vi "Module for RF and LO synthesizer.vi"(10 "Main controller mailbox":T3, 11 "THz module mailbox":T3) -> ()   [LabVIEW 2024, in "THz source modeule.lvlib"]
doc: "Module to set constant frequency or simple frequency sweep on RF (main) synthesizer and offset frequency on LO (folowing) synthesizer.\nKey typedefs: THz_Message for module, THz_Comands enum (Ignore, Initialize, Update, Set parameters, Disconnect, End), THz_Sweeep parameters\n\nComands and responses:\nInitialize: VDI config constants {Master{lower limit, upper limit, name, handle, description}, Follower{ lower limit, upper limit, name, handle, description } } (cluster of two clusters {numeric, numeric, string, numeric, string}) / handle log (string)\nUpdate: - / M_ID F_ID (string)\nSet parameters: Sweep parameters {Start, End, Sweep up time, Sweep down time, Intermediate, Reset trigger} (cluster{numeric, numeric, numeric, numeric, numeric, boolean}) / Sweep parameters (same cluster)\nDisconnect: - / master and follower name (string)\nEnd: - / Master and Follower handle (string)"
uses:
  THz source modeule.lvlib
  Messenger service/Data types/Mailbox address.ctl
  ctl/THz MW generator constants.ctl
  ctl/THz sweep parameters.ctl
  Messenger service/Data types/Module name.ctl
  ctl/THz Message for module.ctl
  ctl/THz commands enum.ctl
  <vilib>/Utility/error.llb/Error Cluster From Error Code.vi
  <vilib>/ErrorRing/Error Ring.xnode
  Messenger service/MessengerLib.lvlib
panel:
  out "FT_Status_Update_Master":u32(ring) items=["FT_OK", "FT_INVALID_HANDLE", "FT_DEVICE_NOT_FOUND", "FT_DEVICE_NOT_OPENED", "FT_IO_ERROR", "FT_INSUFFICIENT_RESOURCES", "FT_INVALID_PARAMETER", "FT_INVALID_BAUD_RATE", "FT_DEVICE_NOT_OPENED_FOR_ERASE", "FT_DEVICE_NOT_OPENED_FOR_WRITE", "FT_FAILED_TO_WRITE_DEVICE", "FT_EEPROM_READ_FAILED", "FT_EEPROM_WRITE_FAILED", "FT_EEPROM_ERASE_FAILED", "FT_EEPROM_NOT_PRESENT", "FT_EEPROM_NOT_PROGRAMMED", "FT_INVALID_ARGS", "FT_NOT_SUPPORTED", "FT_OTHER_ERROR"]
  out "Sweep parameters":T1={"Start [GHz]"=8.0, "End [GHz] "=8.0, "Sweep up\ntime [ms]"=0.0, "Sweep down\ntime [ms]"=0.0, "Intermidiate [MHz]"=0.0, "Reset trigger"=FALSE} {"Sweep down\ntime [ms]" min=0.0 max=250.0; "End [GHz]" min=8.0 max=20.0; "Intermidiate [MHz]" min=0.0 max=2500.0; "Start [GHz]" min=8.0 max=20.0}
  out "FT_Status Update F":u32(ring) items=["FT_OK", "FT_INVALID_HANDLE", "FT_DEVICE_NOT_FOUND", "FT_DEVICE_NOT_OPENED", "FT_IO_ERROR", "FT_INSUFFICIENT_RESOURCES", "FT_INVALID_PARAMETER", "FT_INVALID_BAUD_RATE", "FT_DEVICE_NOT_OPENED_FOR_ERASE", "FT_DEVICE_NOT_OPENED_FOR_WRITE", "FT_FAILED_TO_WRITE_DEVICE", "FT_EEPROM_READ_FAILED", "FT_EEPROM_WRITE_FAILED", "FT_EEPROM_ERASE_FAILED", "FT_EEPROM_NOT_PRESENT", "FT_EEPROM_NOT_PROGRAMMED", "FT_INVALID_ARGS", "FT_NOT_SUPPORTED", "FT_OTHER_ERROR"]
  out "Ended":bool
  out "Constants":T2[](array[typedef])=[{"Lower limit [GHz]"=9.0, "Upper limit [GHz]"=15.0, "Device name"="VDIS0122", "Connection"="0", "Description"="VDI Synth", "Connected"=FALSE, "Last settings"="", "Operation mode"=enum."Disabled", "Enable ch 1"=FALSE, "Enable ch 2"=FALSE}, {"Lower limit [GHz]"=0.01, "Upper limit [GHz]"=1.3, "Device name"="VDIYT7", "Connection"="0", "Description"="VDI Tracking", "Connected"=FALSE, "Last settings"="", "Operation mode"=enum."Disabled", "Enable ch 1"=FALSE, "Enable ch 2"=FALSE}]
  out "Connected":bool
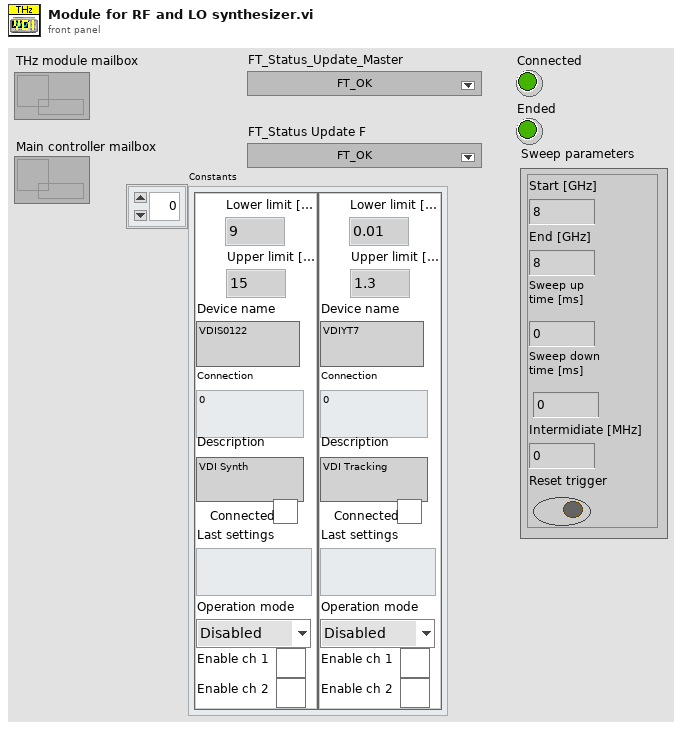
[diagram p1: front panel]
types:
  T1 = typedef "THz source modeule.lvlib/THz sweep parameters.ctl" = cluster{"Start [GHz]":dbl, "End [GHz] ":dbl, "Sweep up\ntime [ms]":dbl, "Sweep down\ntime [ms]":dbl, "Intermidiate [MHz]":dbl, "Reset trigger":bool}
  T2 = typedef "THz source modeule.lvlib/THz MW generator constants.ctl" = cluster{"Lower limit [GHz]":dbl, "Upper limit [GHz]":dbl, "Device name":string, "Connection":string, "Description":string, "Connected":bool, "Last settings":string, "Operation mode":enum16{"Disabled", "CW", "Arbitrary", "Sweep"}, "Enable ch 1":bool, "Enable ch 2":bool}
  T3 = typedef "MessengerLib.lvlib/Mailbox address.ctl" = refnum<queue>
  T4 = typedef "THz source modeule.lvlib/THz Message for module.ctl" = cluster{"Command":T5, "Data":variant}
  T5 = typedef "THz source modeule.lvlib/THz commands enum.ctl" = enum16{"Ignore", "Connect", "Update", "Set parameters", "Disconnect", "End"}
  T6 = typedef "Module name.ctl" = enum16{"Emty", "Magnet", "VTI", "Excitation", "Servo", "Acquisition", "Rotator", "Digitizer", "SMU2450", "Carousel", "Multimeter", "Tmp monitor", "Power monitor"}
  T7 = typedef "THz source modeule.lvlib/VDI status.ctl" = cluster{"Master":T8, "Follower":T8}
  T8 = typedef "THz source modeule.lvlib/Synth status.ctl" = cluster{"Mode":enum16{"CW", "Sweep"}, "Conected":bool}
  T9 = cluster{"Type":u32, "VID":string, "PID":string, "Serial Number":string, "Description":string}
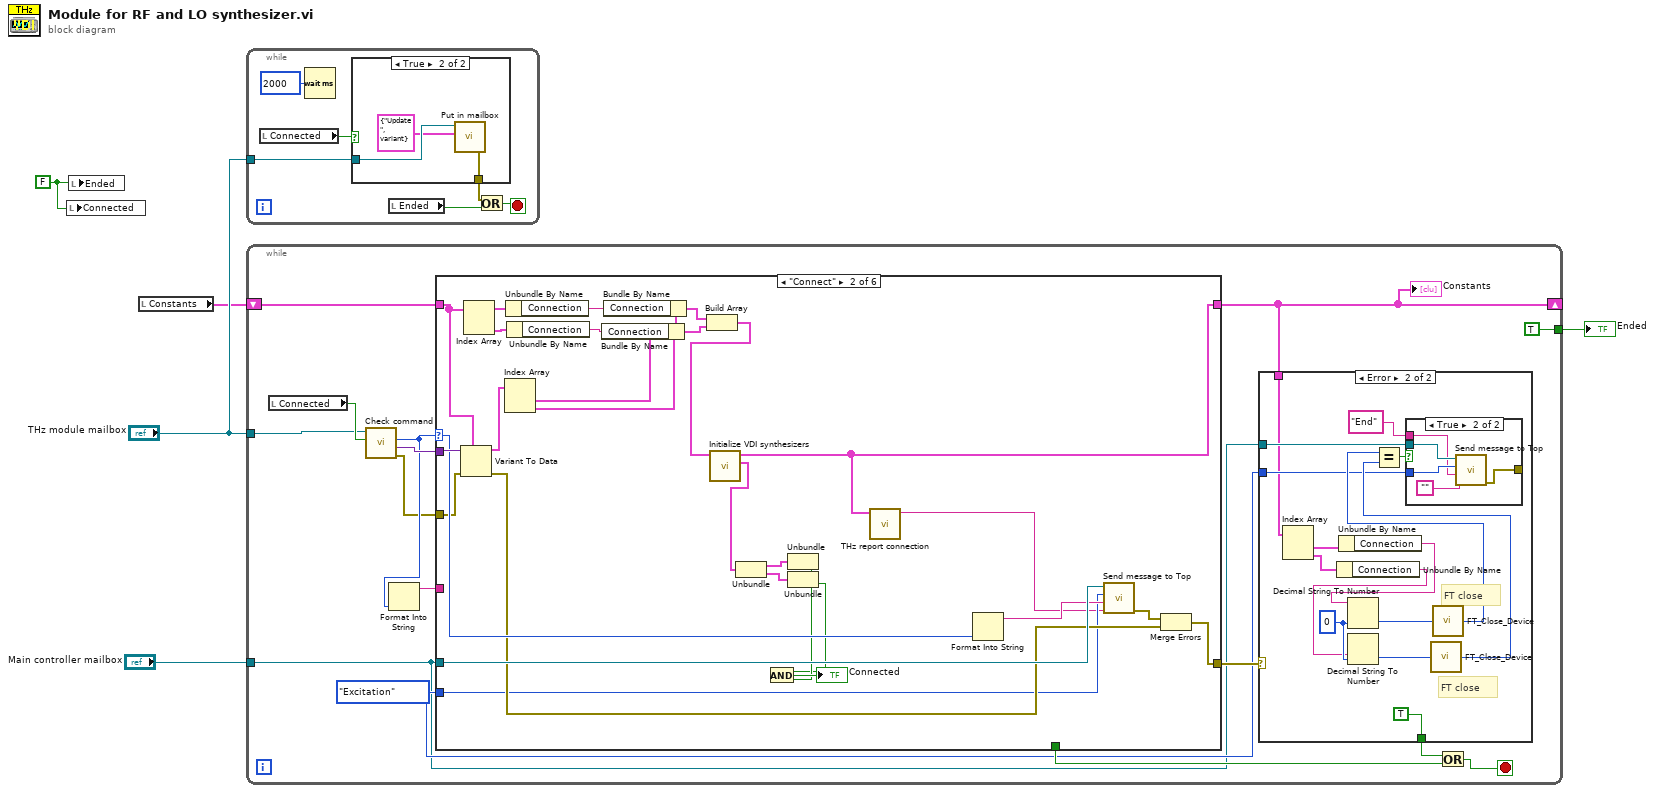
[diagram p0: block diagram]
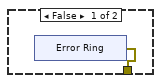
[diagram p2: hidden frame]
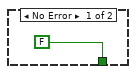
[diagram p3: hidden frame]
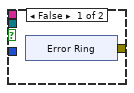
[diagram p4: hidden frame]
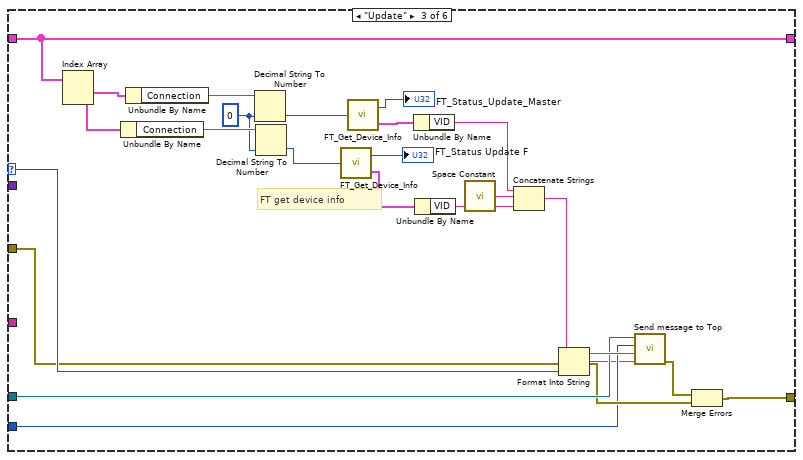
[diagram p6: hidden frame]
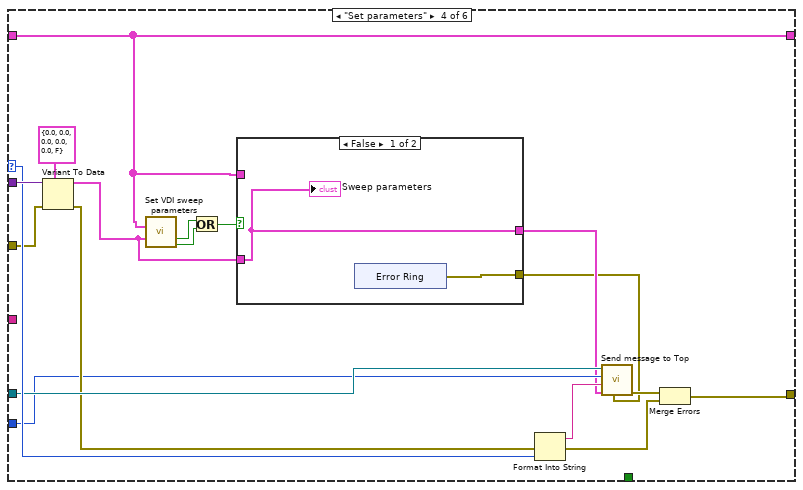
[diagram p7: hidden frame]
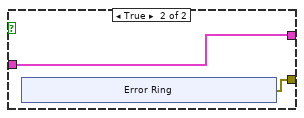
[diagram p8: hidden frame]
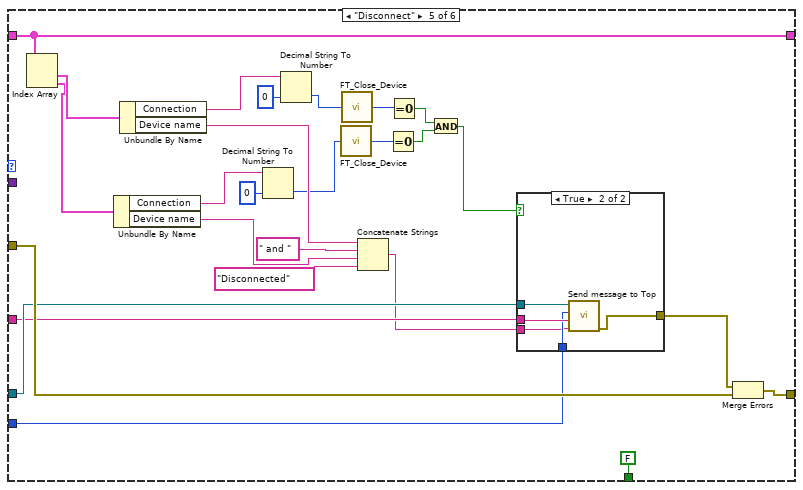
[diagram p9: hidden frame]
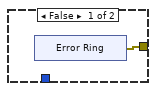
[diagram p10: hidden frame]
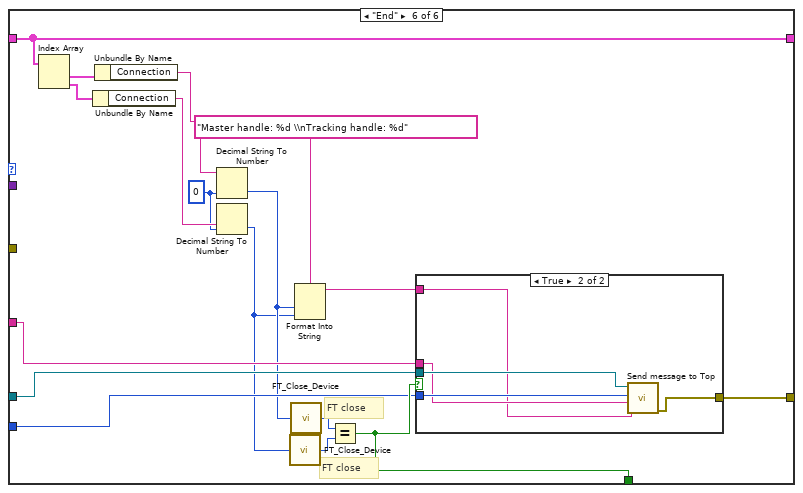
[diagram p11: hidden frame]
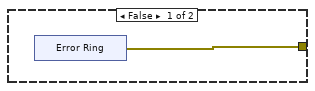
[diagram p12: hidden frame]
diagram:
  w1 = FALSE ("Initialized")
  n1 = local write "Connected"(w1) -> ()
  n2 = local write "Ended"(w1) -> ()
  n3 = local read "Constants"() -> (w3:T2[])
  n4 = while {
    tunnel: "THz module mailbox" -> [w9]
    stop <- w8 stop-if-true
    n5 = local read "Connected"() -> (w10:bool)
    n6 = Wait (ms)(milliseconds to wait=u32 2000) -> ()  [unwired: 1 out]
    n7 = case shown="True" w10 {
      tunnel: w9 -> [_ w16]
      tunnel: [w12 w14] -> w7
      frame False {
        n8 = xnode "Error Ring"() -> ("error out"=w12:errorcluster)
      }
      frame True {
        n9 = call "Put in mailbox.vi"("Message"=T4 {"Command"=enum."Update", "Data"=variant} ("Incoming msg"), "Queue in"=w16) -> ("error out"=w14:errorcluster)  [unwired: 7 in, 2 out]
      }
    }
    n10 = local read "Ended"() -> (w6:bool)
    n11 = Or(x=w7, y=w6) -> (x .or. y?=w8:bool)
  }
  n12 = while {
    shift-right: [w28] -> _
    shift-left: w3 -> [w31]
    tunnel: "THz module mailbox" -> [w20]
    tunnel: "Main controller mailbox" -> [w17]
    tunnel: [TRUE ("Initialized")] -> w2
    stop <- w26 stop-if-true
    w18 = Module_name."Excitation" ("Module")
    n13 = local read "Connected"() -> (w29:bool)
    n14 = call "Check command.vi"("Is connected"=w29, "Module mailbox"=w20) -> ("error out"=w19:errorcluster, "Command Data"=w30:variant, "Command"=w22:T5)  [unwired: 3 in]
    n15 = Format Into String(w22) -> (resulting string=w21:string)  [unwired: 3 in, 1 out]
    n16 = case shown="\"Connect\"" w22 {
      selector: w22 -> [_ w83 w107 w123 _ _]
      tunnel: [w56 w58 w101 w109 w158 w172] -> w28
      tunnel: w31 -> [w56 w71 w101 w109 w158 w172]
      tunnel: w30 -> [_ w84 _ w126 _ _]
      tunnel: [_ _ _ _ FALSE w184] -> w27
      tunnel: w17 -> [_ w82 w106 w121 w157 w185]
      tunnel: [w55 w78 w104 w117 w160 w183] -> w23
      tunnel: w19 -> [w55 w76 w103 w119 w161 _]
      tunnel: w18 -> [_ w72 w100 w114 w150 w179]
      tunnel: w21 -> [_ _ _ _ w151 w182]
      frame "Ignore", Default {
      }
      frame "Connect" {
        n17 = Variant To Data(error in=w76, type=w71, Variant=w84) -> (data=w68:T2[], error out=w75:errorcluster)
        n18 = Index Array(array=w71) -> (element #1=w70:T2, element #2=w69:T2)  [unwired: 2 in]
        n19 = Index Array(array=w68) -> (element #1=w67:T2, element #2=w63:T2)  [unwired: 2 in]
        n20 = Unbundle By Name(w70) -> ("Connection"=w66:string)
        n21 = Unbundle By Name(w69) -> ("Connection"=w61:string)
        n22 = Bundle By Name(cluster=w63, "Connection"=w61) -> (w62:T2)
        n23 = Bundle By Name(cluster=w67, "Connection"=w66) -> (w64:T2)
        n24 = Build Array(w64, w62) -> (w65:T2[])
        n25 = call "Initialize VDI synthesizers.vi"("VDI config constants in"=w65) -> ("Status"=w74:T7, "VDI config constants out"=w58:T2[])  [unwired: 9 in]
        n26 = Unbundle(w74) -> ("Master"=w79:T8, "Follower"=w73:T8)
        n27 = Unbundle(w79) -> ("Conected"=w60:bool)  [unwired: 1 out]
        n28 = Unbundle(w73) -> ("Conected"=w59:bool)  [unwired: 1 out]
        n29 = And(x=w59, y=w60) -> (x .and. y?=→"Connected":bool)
        n30 = call "THz report connection.vi"("THz MW generator constants"=w58) -> ("string out"=w57:string)  [unwired: 10 in]
        n31 = Format Into String(w83) -> (resulting string=w81:string)  [unwired: 3 in, 1 out]
        n32 = call "Send message to Top.vi"("Data"=w57, "Response"=w81, "Module"=w72, "Mailbox address in"=w82) -> ("Error out"=w77:errorcluster)  [unwired: 6 in, 1 out]
        n33 = Merge Errors(w77, w75) -> (w78:errorcluster)
      }
      frame "Update" {
        w87 = u32 0 ("default (0 I32)")
        # "FT get device info"
        n34 = Index Array(array=w101) -> (element #1=w88:T2, element #2=w89:T2)  [unwired: 2 in]
        n35 = Unbundle By Name(w89) -> ("Connection"=w90:string)
        n36 = Unbundle By Name(w88) -> ("Connection"=w91:string)
        n37 = Decimal String To Number(string=w91, default (0L)=w87) -> (number=w86:u32)  [unwired: 1 in, 1 out]
        n38 = Decimal String To Number(string=w90, default (0L)=w87) -> (number=w85:u32)  [unwired: 1 in, 1 out]
        n39 = call <instrlib>:"FT_Get_Device_Info.vi"("Handle"=w85) -> ("FT_Status"=→"FT_Status Update F":u32, "Device Information"=w99:T9)
        n40 = call <instrlib>:"FT_Get_Device_Info.vi"("Handle"=w86) -> ("FT_Status"=→"FT_Status_Update_Master":u32, "Device Information"=w97:T9)
        n41 = Unbundle By Name(w97) -> ("VID"=w95:string)
        n42 = Unbundle By Name(w99) -> ("VID"=w98:string)
        n43 = call <vilib>:"Space Constant.vi"() -> ("String"=w94:string)
        n44 = Concatenate Strings(w95, w94, w98) -> (w96:string)
        n45 = Format Into String(error in=w103, w107) -> (resulting string=w108:string, error out=w102:errorcluster)  [unwired: 2 in]
        n46 = call "Send message to Top.vi"("Data"=w96, "Response"=w108, "Module"=w100, "Mailbox address in"=w106) -> ("Error out"=w105:errorcluster)  [unwired: 6 in, 1 out]
        n47 = Merge Errors(w105, w102) -> (w104:errorcluster)
      }
      frame "Set parameters" {
        n48 = Variant To Data(error in=w119, type=T1 {"Start [GHz]"=0.0, "End [GHz] "=0.0, "Sweep up\ntime [ms]"=0.0, "Sweep down\ntime [ms]"=0.0, "Intermidiate [MHz]"=0.0, "Reset trigger"=FALSE} ("Sweep parameters"), Variant=w126) -> (data=w111:T1, error out=w118:errorcluster)
        n49 = call "Set VDI sweep parameters.vi"("MW generator constants"=w109, "Sweep parameters"=w111) -> ("Error1"=w122:bool, "Error2"=w120:bool)  [unwired: 9 in, 3 out]
        n50 = Or(x=w122, y=w120) -> (x .or. y?=w113:bool)
        n51 = case shown="False" w113 {
          tunnel: [w128 w130] -> w112
          tunnel: w111 -> [w128 w130]
          tunnel: w109 -> [_ _]
          tunnel: [w127 w131] -> w110
          frame False {
            n52 = xnode "Error Ring"() -> ("error out"=w127:errorcluster)
            "Sweep parameters" <- w128
          }
          frame True {
            n53 = xnode "Error Ring"() -> ("error out"=w131:errorcluster)
          }
        }
        n54 = Format Into String(error in=w118, w123) -> (resulting string=w124:string, error out=w116:errorcluster)  [unwired: 2 in]
        n55 = call "Send message to Top.vi"("Error in (no error)"=w110, "Data"=w112, "Response"=w124, "Module"=w114, "Mailbox address in"=w121) -> ("Error out"=w115:errorcluster)  [unwired: 5 in, 1 out]
        n56 = Merge Errors(w115, w116) -> (w117:errorcluster)
      }
      frame "Disconnect" {
        n57 = Index Array(array=w158) -> (element #1=w143:T2, element #2=w141:T2)  [unwired: 2 in]
        n58 = Unbundle By Name(w141) -> ("Connection"=w136:string, "Device name"=w142:string)
        n59 = Unbundle By Name(w143) -> ("Connection"=w159:string, "Device name"=w149:string)
        n60 = Decimal String To Number(string=w136, default (0L)=u32 0 ("default (0 I32)")) -> (number=w137:u32)  [unwired: 1 in, 1 out]
        n61 = Decimal String To Number(string=w159, default (0L)=u32 0 ("default (0 I32)")) -> (number=w140:u32)  [unwired: 1 in, 1 out]
        n62 = call <instrlib>:"FT_Close_Device.vi"("Handle"=w137) -> ("FT_Status"=w155:u32)
        n63 = call <instrlib>:"FT_Close_Device.vi"("Handle"=w140) -> ("FT_Status"=w154:u32)
        n64 = Concatenate Strings(w149, " and " ("string"), w142, "Disconnected" ("string")) -> (w144:string)
        n65 = Equal To 0?(x=w155) -> (x = 0?=w156:bool)
        n66 = Equal To 0?(x=w154) -> (x = 0?=w153:bool)
        n67 = And(x=w153, y=w156) -> (x .and. y?=w152:bool)
        n68 = case shown="True" w152 {
          tunnel: w157 -> [_ w168]
          tunnel: [w162 w167] -> w146
          tunnel: w151 -> [_ w166]
          tunnel: w150 -> [_ w165]
          tunnel: w144 -> [_ w164]
          frame False {
            n69 = xnode "Error Ring"() -> ("error out"=w162:errorcluster)
          }
          frame True {
            n70 = call "Send message to Top.vi"("Data"=w164, "Response"=w166, "Module"=w165, "Mailbox address in"=w168) -> ("Error out"=w167:errorcluster)  [unwired: 6 in, 1 out]
          }
        }
        n71 = Merge Errors(w146, w161) -> (w160:errorcluster)
      }
      frame "End" {
        w173 = u32 0 ("default (0 I32)")
        # "FT close"
        # "FT close"
        n72 = Index Array(array=w172) -> (element #1=w174:T2, element #2=w175:T2)  [unwired: 2 in]
        n73 = Unbundle By Name(w175) -> ("Connection"=w176:string)
        n74 = Unbundle By Name(w174) -> ("Connection"=w171:string)
        n75 = Decimal String To Number(string=w171, default (0L)=w173) -> (number=w170:u32)  [unwired: 1 in, 1 out]
        n76 = Decimal String To Number(string=w176, default (0L)=w173) -> (number=w169:u32)  [unwired: 1 in, 1 out]
        n77 = call <instrlib>:"FT_Close_Device.vi"("Handle"=w169) -> ("FT_Status"=w180:u32)
        n78 = call <instrlib>:"FT_Close_Device.vi"("Handle"=w170) -> ("FT_Status"=w181:u32)
        n79 = Format Into String(format string="Master handle: %d \\nTracking handle: %d", w170, w169) -> (resulting string=w177:string)  [unwired: 2 in, 1 out]
        n80 = Equal?(x=w181, y=w180) -> (x = y?=w184:bool)
        n81 = case shown="True" w184 {
          tunnel: w185 -> [_ w192]
          tunnel: [w186 w191] -> w183
          tunnel: w179 -> [_ w190]
          tunnel: w182 -> [_ w189]
          tunnel: w177 -> [_ w188]
          frame False {
            n82 = xnode "Error Ring"() -> ("error out"=w186:errorcluster)
          }
          frame True {
            n83 = call "Send message to Top.vi"("Data"=w188, "Response"=w189, "Module"=w190, "Mailbox address in"=w192) -> ("Error out"=w191:errorcluster)  [unwired: 6 in, 1 out]
          }
        }
      }
    }
    "Constants" <- w28
    n84 = case shown="Error" w23 {
      tunnel: w28 -> [_ w40]
      tunnel: [FALSE TRUE] -> w25
      tunnel: w18 -> [_ w42]
      tunnel: w17 -> [_ w41]
      frame No Error {
      }
      frame Error {
        w39 = u32 0 ("default (0 I32)")
        # "FT close"
        # "FT close"
        n85 = Index Array(array=w40) -> (element #1=w38:T2, element #2=w37:T2)  [unwired: 2 in]
        n86 = Unbundle By Name(w37) -> ("Connection"=w36:string)
        n87 = Unbundle By Name(w38) -> ("Connection"=w35:string)
        n88 = Decimal String To Number(string=w35, default (0L)=w39) -> (number=w34:u32)  [unwired: 1 in, 1 out]
        n89 = Decimal String To Number(string=w36, default (0L)=w39) -> (number=w33:u32)  [unwired: 1 in, 1 out]
        n90 = call <instrlib>:"FT_Close_Device.vi"("Handle"=w33) -> ("FT_Status"=w43:u32)
        n91 = call <instrlib>:"FT_Close_Device.vi"("Handle"=w34) -> ("FT_Status"=w44:u32)
        n92 = Equal?(x=w44, y=w43) -> (x = y?=w46:bool)
        n93 = case shown="True" w46 {
          tunnel: w41 -> [_ w54]
          tunnel: [w48 w53] -> _
          tunnel: w42 -> [_ w51]
          tunnel: "End" -> [_ w50]
          frame False {
            n94 = xnode "Error Ring"() -> ("error out"=w48:errorcluster)
          }
          frame True {
            n95 = call "Send message to Top.vi"("Data"="", "Response"=w50, "Module"=w51, "Mailbox address in"=w54) -> ("Error out"=w53:errorcluster)  [unwired: 6 in, 1 out]
          }
        }
      }
    }
    n96 = Or(x=w25, y=w27) -> (x .or. y?=w26:bool)
  }
  "Ended" <- w2
